vi "ManuBarcodetest.vi"(11 "String":string) -> (2 "x = y?":bool, 3 "before substring":string)   [LabVIEW 2014]
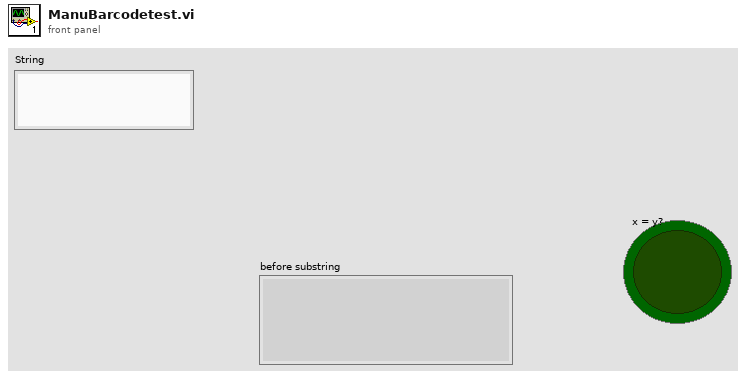
[diagram p1: front panel]
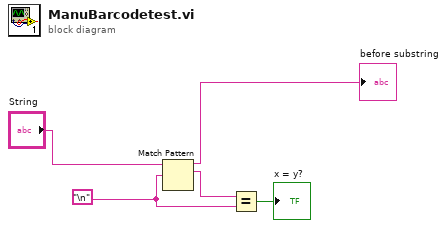
[diagram p0: block diagram]
diagram:
  w2 = "\n"
  n1 = Match Pattern(string="String", regular expression=w2) -> (before substring=→"before substring":string, match substring=w5:string)  [unwired: 1 in, 2 out]
  n2 = Equal?(x=w5, y=w2) -> (x = y?=→"x = y?":bool)
